vi "tsapp_check_lin_channel_is_ready.vi"(8 "错误输入（无错误）":errorcluster, 10 "AAppChnIndex":i32, 11 "路径输入":path) -> (0 "错误输出":errorcluster, 2 "return":i32, 3 "路径输出":path)   [LabVIEW 2014]
doc: "Function Introduction :\nCheck if LIN channel is ready\nCall location :\nAfter mapping the LIN channel, check if the LIN channel is ready according to the application requirements\ninput parameter :\nAAppChnInDex: Channel Index\nReturn value :\n==0: Execution successful\nOther values: Query error code"
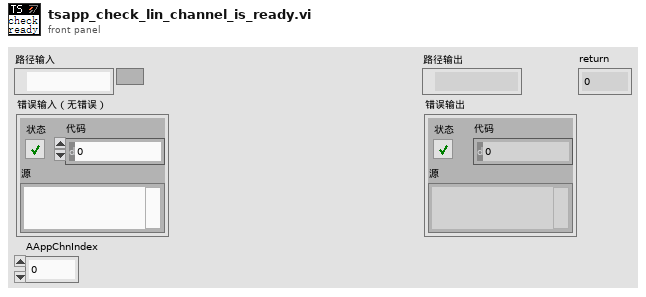
[diagram p1: front panel]
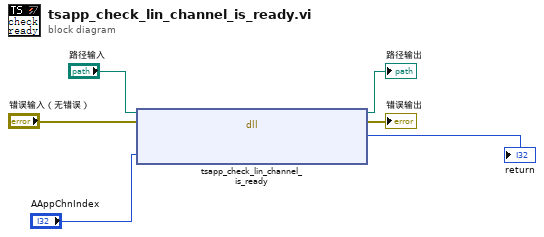
[diagram p0: block diagram]
diagram:
  n1 = dll-call lib="D:/Program Files (x86)/TOSUN/TSMaster/Data/SDK/lib/x86/TSMaster.dll" fn="tsapp_check_lin_channel_is_ready"(path in="路径输入", error in="错误输入（无错误）", "AAppChnIndex"="AAppChnIndex") -> (path out=→"路径输出":path, error out=→"错误输出":errorcluster, "返回类型"=→"return":i32)  [unwired: 2 in]
